vi "Periodic Tasks.vi"() -> ()   [LabVIEW 2012]
doc: "This VI runs in parallel to other tasks. It can contain as many user-defined periodic loops as you need. These can carry out PID or other sorts of timed response."
uses:
  <vilib>/Rock Robotics/SystemInterfaces/Utilities/FPGA_UtilitiesLED Source.ctl
  <vilib>/Rock Robotics/SystemInterfaces/Utilities/FPGA_UtilitiesLED State.ctl
  Robot Global Data.vi
panel:
  in  "FlipUp":bool
  in  "ClimberHooked":bool
  in  "Use DS Data":bool
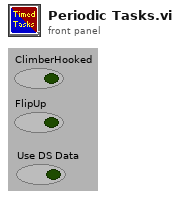
[diagram p1: front panel]
types:
  T1 = typedef "FPGA_UtilitiesLED State.ctl" = enum16{"Off", "On", "Toggle"}
  T2 = typedef "FPGA_UtilitiesLED Source.ctl" = enum16{"User LED", "FPGA LED"}
  T3 = cluster{"Case":dbl, "VisionTrack":bool, "ShootEnableWheels":bool, "Shoot":bool, "ManualExtend":dbl, "ManualRotate":dbl, "YCoord":dbl, "FlipUp":bool, "RotDeadband":dbl, "ExtDeadband":dbl, "ExtPOT":dbl, "RotPOT":dbl, "WheelFSpd":dbl, "WheelBSpd":dbl, "ServoPositions":cluster{"FlipperLeftUp":dbl, "FlipperLeftDown":dbl, "FlipperRightUp":dbl, "FlipperRightDown":dbl, "KickerLeftBack":dbl, "KickerLeftForward":dbl, "KickerRightBack":dbl, "KickerRightForward":dbl}, "POTPositions":cluster{"Setpoint 1":dbl, "Setpoint 2":dbl, "Setpoint 3":dbl, "Setpoint 4":dbl, "RotLow":dbl, "RotHigh":dbl, "ExtLow":dbl, "ExtHigh":dbl}, "ClimberHooked":bool}
  T4 = cluster{"FlipperLeftUp":dbl, "FlipperLeftDown":dbl, "FlipperRightUp":dbl, "FlipperRightDown":dbl, "KickerLeftBack":dbl, "KickerLeftForward":dbl, "KickerRightBack":dbl, "KickerRightForward":dbl}
  T5 = cluster{"Setpoint 1":dbl, "Setpoint 2":dbl, "Setpoint 3":dbl, "Setpoint 4":dbl, "RotLow":dbl, "RotHigh":dbl, "ExtLow":dbl, "ExtHigh":dbl}
  T6 = typedef "WPI_AnalogChannelDevRef.ctl" = cluster{"DevStatus":errorcluster, "Analog Module":T7, "Analog Channel":T8}
  T7 = typedef "FPGA_TypedefAnalogModule.ctl" = enum16{"Analog Module 1", "Analog Module 2"}
  T8 = typedef "FPGA_AIChannel.ctl" = enum8{"AI 1", "AI 2", "AI 3", "AI 4", "AI 5", "AI 6", "AI 7", "AI 8", "Invalid"}
  T9 = typedef "WPI_GyroDevRef.ctl" = cluster{"DevStatus":errorcluster, "Analog Module":T7, "Analog Channel":T8, "Offset":dbl, "Gain (VoltsPerDegree/Second)":dbl}
  T10 = typedef "WPI_EncoderDevRef.ctl" = cluster{"DevStatus":errorcluster, "EncoderIndex":T11, "CounterIndex":T12, "DistancePerCount":dbl, "Decoding Type":T13}
  T11 = typedef "FPGA_EncoderIdx.ctl" = enum8{"Enc 0", "Enc 1", "Enc 2", "Enc 3", "Invalid"}
  T12 = typedef "FPGA_CounterCtrSystemIndex.ctl" = enum8{"Ctr 0", "Ctr 1", "Ctr 2", "Ctr 3", "Ctr 4", "Ctr 5", "Ctr 6", "Ctr 7", "Invalid"}
  T13 = typedef "WPI_EncoderType.ctl" = enum16{"1x", "2x", "4x"}
  T14 = typedef "WPI_RelayValue.ctl" = enum16{"Off", "On", "Forward", "Reverse"}
  T15 = cluster{"Case":dbl, "Extension":dbl, "Rotation":dbl, "WheelF":dbl, "WheelB":dbl, "Left Kicker":dbl, "Right Kicker":dbl, "Left Flipper":dbl, "Right Flipper":dbl, "Lights":T14}
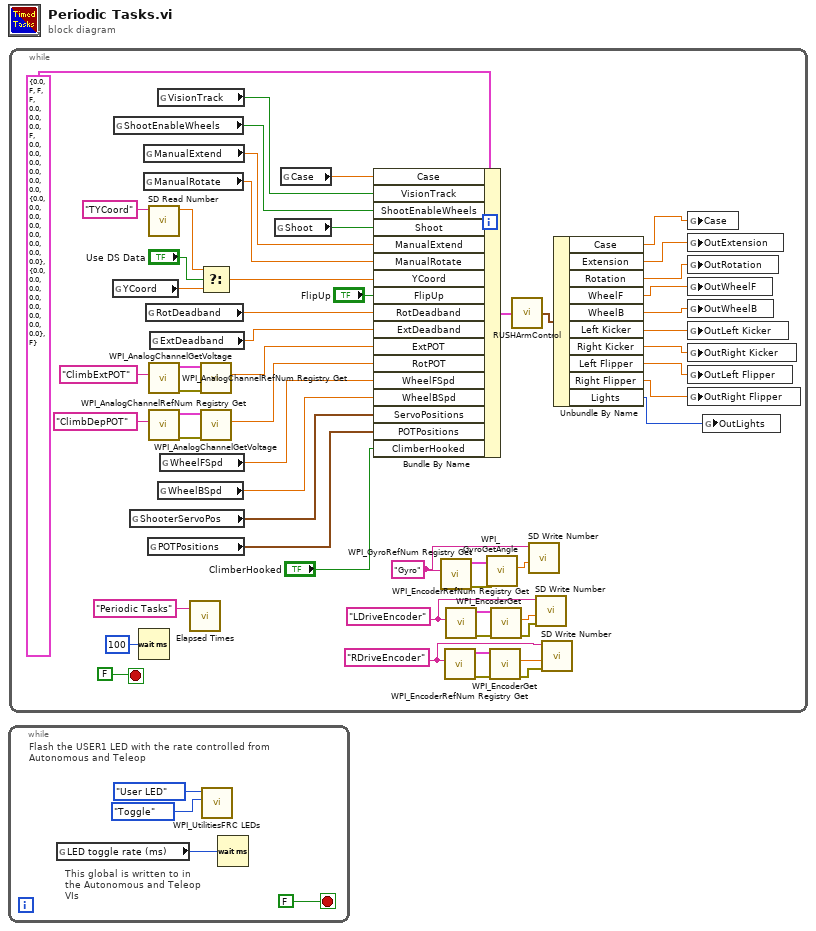
[diagram p0: block diagram]
diagram:
  n1 = while {
    stop <- FALSE stop-if-true
    # "This global is written to in the Autonomous and Teleop VIs"
    # "Flash the USER1 LED with the rate controlled from Autonomous and Teleop"
    n2 = global read "Robot Global Data.vi" "LED toggle rate (ms)"() -> (w1:u32)
    n3 = call <vilib>:"WPI_UtilitiesFRC LEDs.vi"("State"=FPGA_UtilitiesLED_State."Toggle", "LED Type"=FPGA_UtilitiesLED_Source."User LED") -> ()  [unwired: 1 in, 9 out]
    n4 = Wait (ms)(milliseconds to wait=w1) -> ()  [unwired: 1 out]
  }
  n5 = while {
    stop <- FALSE stop-if-true
    w12 = "RDriveEncoder" ("refnum name")
    w8 = "LDriveEncoder" ("refnum name")
    w6 = "Gyro" ("refnum name")
    n6 = global read "Robot Global Data.vi" "YCoord"() -> (w27:dbl)
    n7 = global read "Robot Global Data.vi" "ShootEnableWheels"() -> (w42:bool)
    n8 = global read "Robot Global Data.vi" "ShooterServoPos"() -> (w34:T4)
    n9 = Wait (ms)(milliseconds to wait=u32 100) -> ()  [unwired: 1 out]
    n10 = global read "Robot Global Data.vi" "ManualExtend"() -> (w40:dbl)
    n11 = global read "Robot Global Data.vi" "ManualRotate"() -> (w39:dbl)
    n12 = global read "Robot Global Data.vi" "RotDeadband"() -> (w38:dbl)
    n13 = global read "Robot Global Data.vi" "POTPositions"() -> (w33:T5)
    n14 = call <vilib>:"SD Read Number.vi"("Name"="TYCoord") -> ("Numeric"=w28:dbl)  [unwired: 8 in, 2 out]
    n15 = call <vilib>:"WPI_AnalogChannelRefNum Registry Get.vi"("refnum name"="ClimbExtPOT") -> ("error out"=w56:errorcluster, "AIDeviceRef"=w55:T6)  [unwired: 9 in]
    n16 = call <vilib>:"WPI_AnalogChannelRefNum Registry Get.vi"("refnum name"="ClimbDepPOT") -> ("error out"=w50:errorcluster, "AIDeviceRef"=w49:T6)  [unwired: 9 in]
    n17 = global read "Robot Global Data.vi" "ExtDeadband"() -> (w37:dbl)
    n18 = global read "Robot Global Data.vi" "VisionTrack"() -> (w43:bool)
    n19 = global read "Robot Global Data.vi" "WheelBSpd"() -> (w35:dbl)
    n20 = global read "Robot Global Data.vi" "WheelFSpd"() -> (w36:dbl)
    n21 = call "Elapsed Times.vi"("Call Name"="Periodic Tasks") -> ()  [unwired: 2 in, 1 out]
    n22 = Select(t=w28, s="Use DS Data", f=w27) -> (s? t:f=w25:dbl)
    n23 = call <vilib>:"WPI_AnalogChannelGetVoltage.vi"("error in (no error)"=w56, "AIDeviceRef"=w55) -> ("Voltage"=w30:dbl)  [unwired: 7 in, 2 out]
    n24 = call <vilib>:"WPI_AnalogChannelGetVoltage.vi"("error in (no error)"=w50, "AIDeviceRef"=w49) -> ("Voltage"=w29:dbl)  [unwired: 7 in, 2 out]
    n25 = global read "Robot Global Data.vi" "Shoot"() -> (w41:bool)
    n26 = global read "Robot Global Data.vi" "Case"() -> (w44:dbl)
    n27 = Bundle By Name(cluster=T3 {"Case"=0.0, "VisionTrack"=FALSE, "ShootEnableWheels"=FALSE, "Shoot"=FALSE, "ManualExtend"=0.0, "ManualRotate"=0.0, "YCoord"=0.0, "FlipUp"=FALSE, "RotDeadband"=0.0, "ExtDeadband"=0.0, "ExtPOT"=0.0, "RotPOT"=0.0, "WheelFSpd"=0.0, "WheelBSpd"=0.0, "ServoPositions"={"FlipperLeftUp"=0.0, "FlipperLeftDown"=0.0, "FlipperRightUp"=0.0, "FlipperRightDown"=0.0, "KickerLeftBack"=0.0, "KickerLeftForward"=0.0, "KickerRightBack"=0.0, "KickerRightForward"=0.0}, "POTPositions"={"Setpoint 1"=0.0, "Setpoint 2"=0.0, "Setpoint 3"=0.0, "Setpoint 4"=0.0, "RotLow"=0.0, "RotHigh"=0.0, "ExtLow"=0.0, "ExtHigh"=0.0}, "ClimberHooked"=FALSE} ("In Cluster"), "Case"=w44, "VisionTrack"=w43, "ShootEnableWheels"=w42, "Shoot"=w41, "ManualExtend"=w40, "ManualRotate"=w39, "YCoord"=w25, "FlipUp"="FlipUp", "RotDeadband"=w38, "ExtDeadband"=w37, "ExtPOT"=w30, "RotPOT"=w29, "WheelFSpd"=w36, "WheelBSpd"=w35, "ServoPositions"=w34, "POTPositions"=w33, "ClimberHooked"="ClimberHooked") -> (w46:T3)
    n28 = call <vilib>:"WPI_GyroRefNum Registry Get.vi"("refnum name"=w6) -> ("error out"=w57:errorcluster, "GyroDevRef"=w58:T9)  [unwired: 9 in]
    n29 = call <vilib>:"WPI_EncoderRefNum Registry Get.vi"("refnum name"=w12) -> ("error out"=w52:errorcluster, "EncoderDevRef"=w51:T10)  [unwired: 9 in]
    n30 = call <vilib>:"WPI_EncoderRefNum Registry Get.vi"("refnum name"=w8) -> ("error out"=w53:errorcluster, "EncoderDevRef"=w54:T10)  [unwired: 9 in]
    n31 = call <vilib>:"WPI_GyroGetAngle.vi"("error in (no error)"=w57, "GyroDevRef"=w58) -> ("Angle"=w7:dbl)  [unwired: 6 in, 3 out]
    n32 = call <vilib>:"WPI_EncoderGet.vi"("error in (no error)"=w52, "EncoderDevRef"=w51) -> ("error out"=w9:errorcluster, "Distance"=w13:dbl)  [unwired: 4 in, 4 out]
    n33 = call <vilib>:"WPI_EncoderGet.vi"("error in (no error)"=w53, "EncoderDevRef"=w54) -> ("error out"=w11:errorcluster, "Distance"=w10:dbl)  [unwired: 4 in, 4 out]
    n34 = call "RUSHArmControl.vi"("In Cluster"=w46) -> ("Out Cluster"=w45:T15)
    n35 = call <vilib>:"SD Write Number.vi"("Numeric"=w7, "Name"=w6) -> ()  [unwired: 8 in, 2 out]
    n36 = call <vilib>:"SD Write Number.vi"("error in"=w11, "Numeric"=w10, "Name"=w8) -> ()  [unwired: 7 in, 2 out]
    n37 = call <vilib>:"SD Write Number.vi"("error in"=w9, "Numeric"=w13, "Name"=w12) -> ()  [unwired: 7 in, 2 out]
    n38 = Unbundle By Name(w45) -> ("Case"=w24:dbl, "Extension"=w23:dbl, "Rotation"=w22:dbl, "WheelF"=w21:dbl, "WheelB"=w20:dbl, "Left Kicker"=w19:dbl, "Right Kicker"=w18:dbl, "Left Flipper"=w17:dbl, "Right Flipper"=w16:dbl, "Lights"=w5:T14)
    n39 = global write "Robot Global Data.vi" "Case"(w24) -> ()
    n40 = global write "Robot Global Data.vi" "OutExtension"(w23) -> ()
    n41 = global write "Robot Global Data.vi" "OutRotation"(w22) -> ()
    n42 = global write "Robot Global Data.vi" "OutWheelF"(w21) -> ()
    n43 = global write "Robot Global Data.vi" "OutWheelB"(w20) -> ()
    n44 = global write "Robot Global Data.vi" "OutLeft Kicker"(w19) -> ()
    n45 = global write "Robot Global Data.vi" "OutRight Kicker"(w18) -> ()
    n46 = global write "Robot Global Data.vi" "OutLeft Flipper"(w17) -> ()
    n47 = global write "Robot Global Data.vi" "OutRight Flipper"(w16) -> ()
    n48 = global write "Robot Global Data.vi" "OutLights"(w5) -> ()
  }
